vi "Sensor Interface View.vi"(8 "error in (no error)":errorcluster, 11 "View Model":T1) -> (0 "error out":errorcluster)   [LabVIEW 2017]
doc: "The interface where a user changes the floor location of the Elevator. Simulates the elevator travelling between floors.\n[Covers: UI4]"
uses:
  View Model/Controls/View Model.ctl
  View Model/Controls/Shared Model.ctl
  Error/Controls/Error Model.ctl
  Error/Controls/Error Event.ctl
  Error/Controls/Error Type.ctl
  Configuration/Controls/Config DB Model.ctl
  Configuration/Controls/Config DB Command.ctl
  Configuration/Controls/Config DB Record.ctl
  Controller/Controls/Controller Model.ctl
  Controller/Controls/Elevator Location.ctl
  Controller/Controls/Elevator Direction Event.ctl
  Controller/Controls/Elevator Direction.ctl
  Controller/Controls/Elevator CMD Event.ctl
  Controller/Controls/Elevator Commands.ctl
panel:
  in  "Elevator Position":u16(slide)=1 min=1 max=4 step=1 scale=1.0..4.0
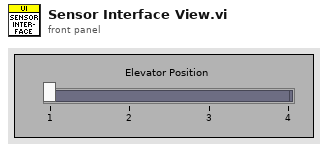
[diagram p1: front panel]
types:
  T1 = typedef "View Model.ctl" = cluster{"Shared Model":T2, "Error Model":T3, "Config Model":T4, "Controller Model":T5}
  T2 = typedef "Shared Model.ctl" = cluster{"Stop":refnum<user-event>, "Stop DVR":refnum<data-value>}
  T3 = typedef "Error Model.ctl" = cluster{"Error":refnum<user-event>}
  T4 = typedef "Config DB Model.ctl" = cluster{"DB Command":refnum<user-event>, "DB Record DVR":refnum<data-value>}
  T5 = typedef "Controller Model.ctl" = cluster{"Go to Floor":refnum<user-event>, "Emergency":refnum<user-event>, "Open/Close Door":refnum<user-event>, "Move To":refnum<user-event>, "Position Change":refnum<user-event>, "Elevator CMD Event":refnum<user-event>}
  T6 = typedef "Elevator Location.ctl" = enum16{"1st Floor", "2nd Floor", "3rd Floor", "4th Floor"}
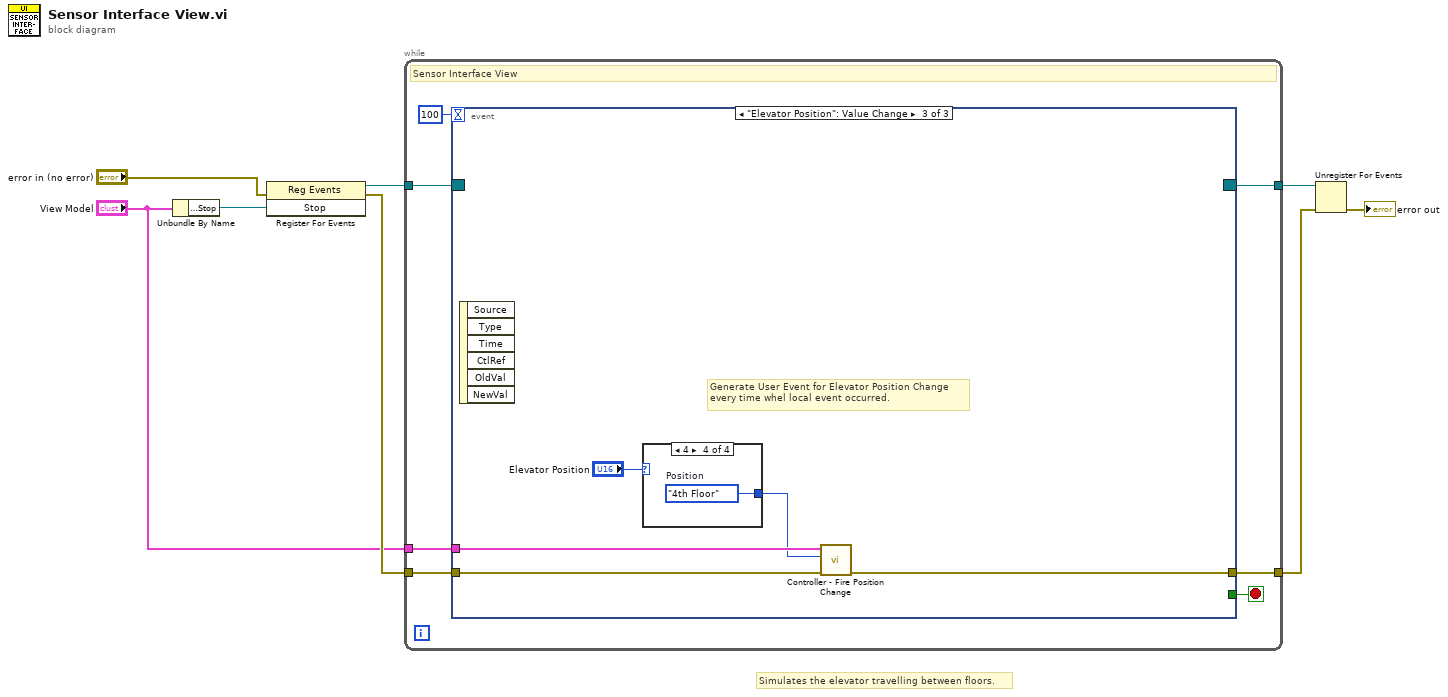
[diagram p0: block diagram]
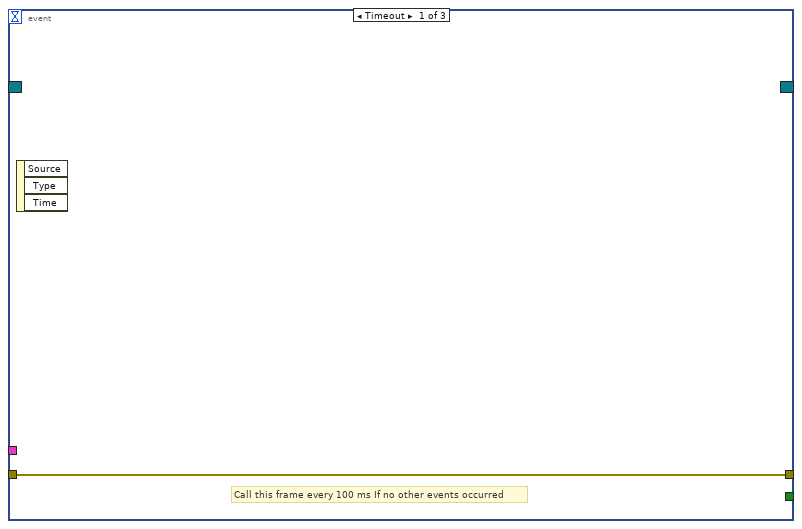
[diagram p2: hidden frame]
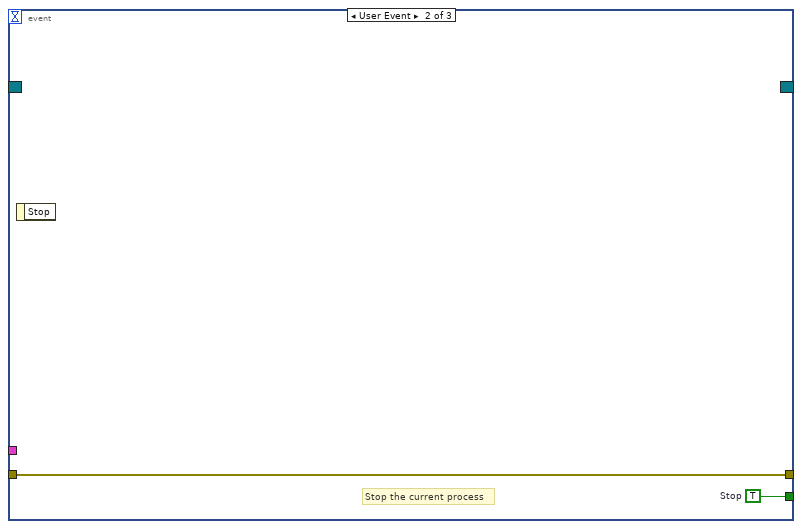
[diagram p3: hidden frame]
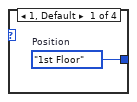
[diagram p4: hidden frame]
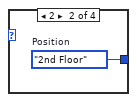
[diagram p5: hidden frame]
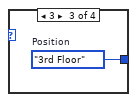
[diagram p6: hidden frame]
diagram:
  # "Simulates the elevator travelling between floors."
  n1 = Unbundle By Name("View Model") -> ("Shared Model.Stop"=w8:refnum<user-event>)
  n2 = register-events(error in="error in (no error)", w8) -> (reference out=w7:refnum<event-registration>, error out=w4:errorcluster)  [unwired: 1 in]
  n3 = while {
    tunnel: w7 -> [w15]
    tunnel: [w14] -> w6
    tunnel: w4 -> [w13]
    tunnel: "View Model" -> [w12]
    tunnel: [w11] -> w2
    stop <- w10 stop-if-true
    # "Sensor Interface View"
    n4 = event shown="[2] \"Elevator Position\": Value Change" {
      selector: w15 -> [_ _ _]
      dyn-events: [_ _ _] -> w14
      timeout: 100 -> [_ _ _]
      tunnel: w13 -> [w16 w18 w22]
      tunnel: w12 -> [_ _ w20]
      tunnel: [w16 w18 w21] -> w11
      tunnel: [_ w17 _] -> w10
      event Timeout {
        # "Call this frame every 100 ms If no other events occurred"
        n5 = event-data() -> ()  [unwired: 1 in, 3 out]
      }
      event User Event {
        w17 = TRUE  # Stop
        # "Stop the current process"
        n6 = event-data() -> ()  [unwired: 1 in, 1 out]
      }
      event "Elevator Position": Value Change {
        # "Generate User Event for Elevator Position Change\nevery time whel local event occurred."
        n7 = event-data() -> ()  [unwired: 1 in, 6 out]
        n8 = case shown="4" "Elevator Position" {
          tunnel: [w24 w25 w26 w27] -> w19
          frame 1, Default {
            w24 = Elevator_Location."1st Floor"  # Position
          }
          frame 2 {
            w25 = Elevator_Location."2nd Floor"  # Position
          }
          frame 3 {
            w26 = Elevator_Location."3rd Floor"  # Position
          }
          frame 4 {
            w27 = Elevator_Location."4th Floor"  # Position
          }
        }
        n9 = call "Controller - Fire Position Change.vi"("error in (no error)"=w22, "Position"=w19, "View Model"=w20) -> ("error out"=w21:errorcluster)  [unwired: 7 in, 1 out]
      }
    }
  }
  n10 = Unregister For Events(event registration refnum=w6, error in=w2) -> (error out=→"error out":errorcluster)
